vi "Script Name Actor.vi"(6 "Name Actor":T1, 8 "error in":errorcluster) -> (0 "error out":errorcluster)   [LabVIEW 2020, in "_Rescript.lvlib" / "Actor.lvlib" / "Actor.lvclass"]
uses:
  Actor.lvclass
  Name Actor.ctl
  Terminal Attributes.ctl
  Attributes.ctl
  Find Pane.vi
  Terminal Attributes Descending Order.vi
  SubVI Terminals.vi
  <vilib>/Utility/traverseref.llb/TRef Find Object By Label.vi
  Script Control To ConPane.vi
  _Rescript.lvlib
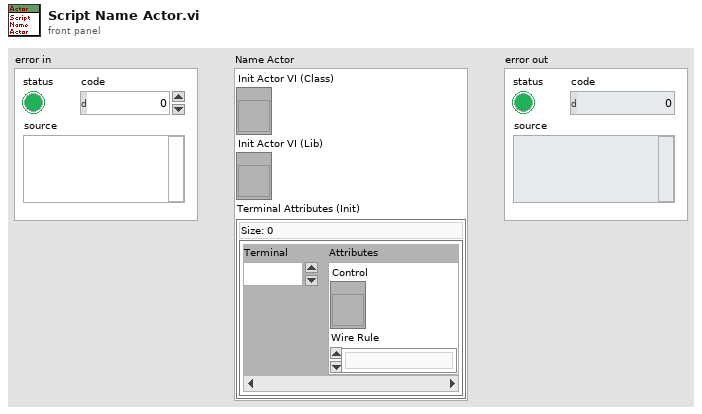
[diagram p1: front panel]
types:
  T1 = typedef "_Rescript.lvlib/Actor.lvlib/Actor.lvclass/Name Actor.ctl" = cluster{"Init Actor VI (Class)":refnum<vi>, "Init Actor VI (Lib)":refnum<vi>, "Terminal Attributes (Init)":T2}
  T2 = typedef "_Rescript.lvlib/Terminal Attributes.ctl" = map{i32, T3}
  T3 = typedef "_Rescript.lvlib/Attributes.ctl" = cluster{"Control":refnum<vi>, "Wire Rule":enum16{"Invalid Wire Rule", "Required", "Recommended", "Optional", "Dynamic Dispatch"}}
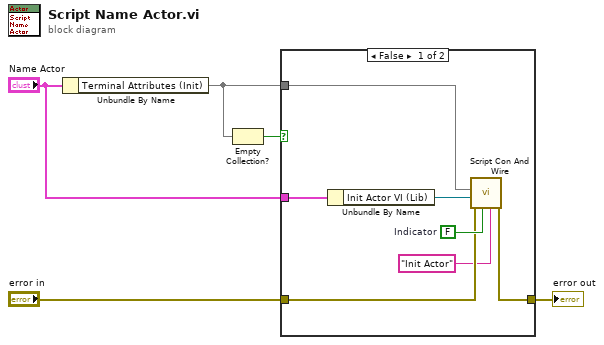
[diagram p0: block diagram]
diagram:
  n1 = Unbundle By Name("Name Actor") -> ("Terminal Attributes (Init)"=w4:T2)
  n2 = Empty Collection?(1:w4) -> (0:w5:bool)
  n3 = case shown="False" w5 {
    tunnel: "error in" -> [w9 w13]
    tunnel: "Name Actor" -> [w10 _]
    tunnel: [w7 w13] -> w2
    tunnel: w4 -> [w6 _]
    frame False {
      w11 = FALSE  # Indicator
      n4 = Unbundle By Name(w10) -> ("Init Actor VI (Lib)"=w12:refnum<vi>)
      n5 = call "Script Con And Wire.vi"("VI Name"="Init Actor" ("format string"), "Indicator"=w11, "error in"=w9, "VI"=w12, "Terminal Attributes"=w6) -> ("error out"=w7:errorcluster)  [unwired: 6 in]
    }
    frame True {
    }
  }
  "error out" <- w2
